vi "user_event_FGV.vi"() -> (3 "bool":refnum<user-event>)   [LabVIEW 2022 SP3]
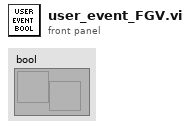
[diagram p1: front panel]
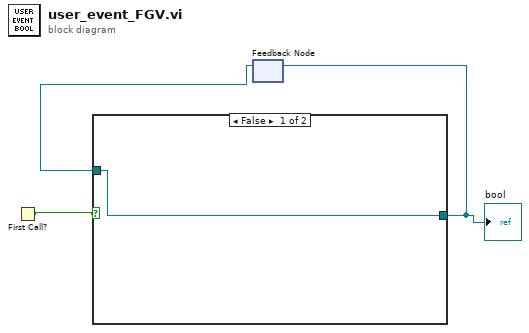
[diagram p0: block diagram]
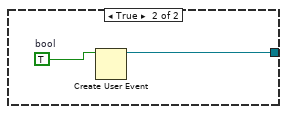
[diagram p2: hidden frame]
diagram:
  n1 = First Call?() -> (First Call?: T/F=w3:bool)
  n2 = feedback #1() -> (w1:refnum<user-event>)  [unwired: 1 in]
  n3 = case shown="False" w3 {
    tunnel: [w4 w5] -> w2
    tunnel: w1 -> [w4 _]
    frame False {
    }
    frame True {
      w6 = TRUE  # bool
      n4 = Create User Event(user event datatype=w6) -> (user event=w5:refnum<user-event>)  [unwired: 1 in, 1 out]
    }
  }
  "bool" <- w2
  n5 = feedback-in #1(w2) -> ()
